vi "PicoLog_DATA.vi"(0 "noOfChannels":i16, 1 "handle":i16, 2 "sampleInterval_ms":dbl) -> (3 "handle":i16, 4 "P4":dbl[](graph), 5 "P5":dbl[](graph), 6 "Waveform Graph 3":dynamicdata(graph), 7 "P1":dbl[](graph), 8 "P2":dbl[](graph), 9 "P3":dbl[](graph))   [LabVIEW 2014]
uses:
  picohrdl.dll
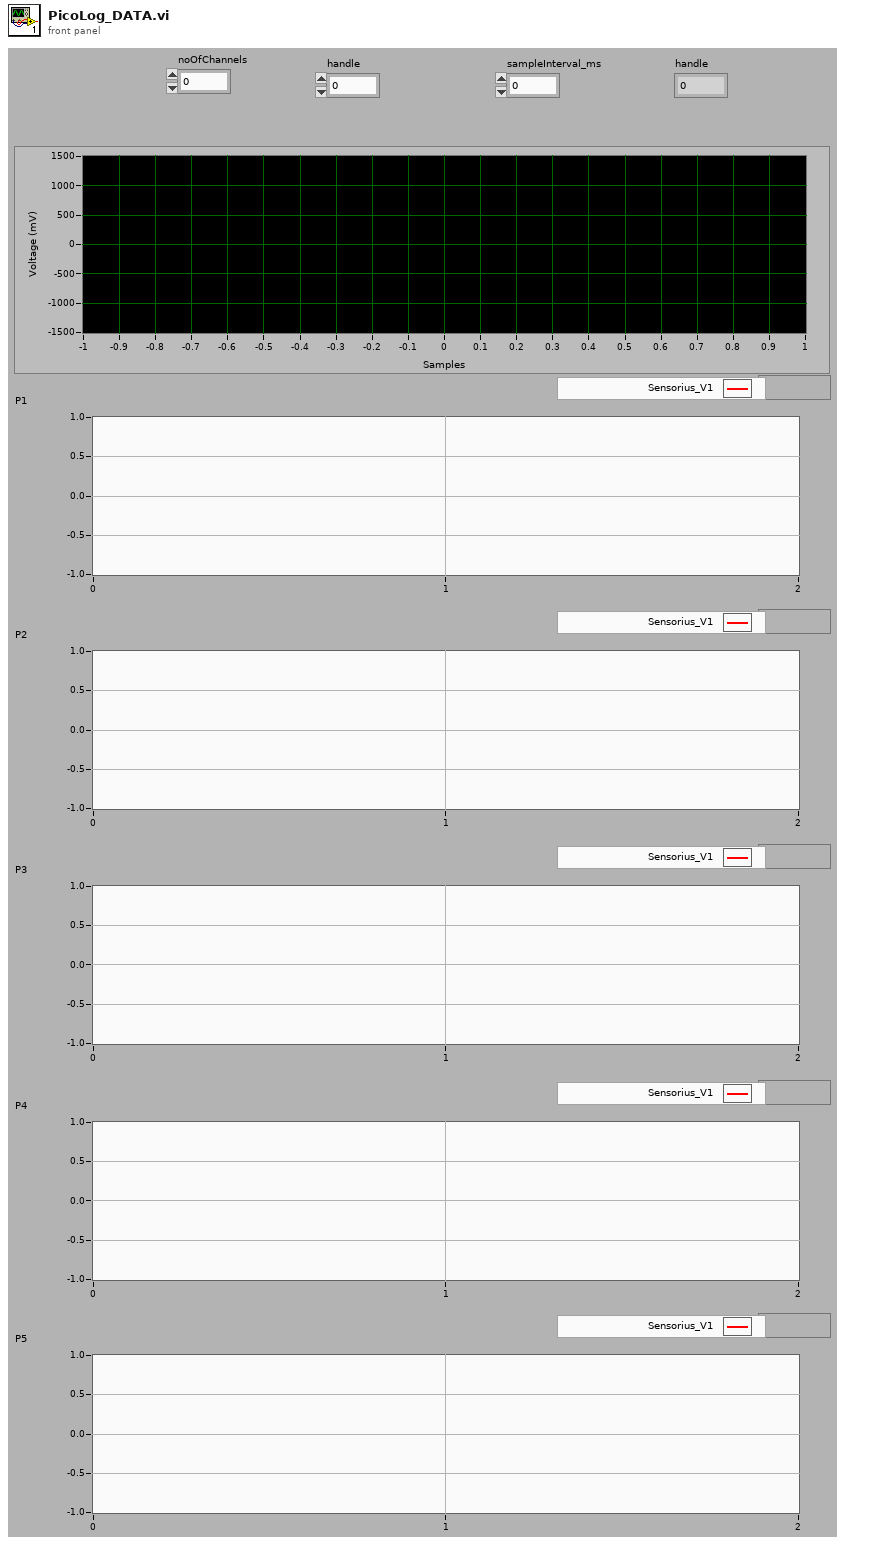
[diagram p1: front panel]
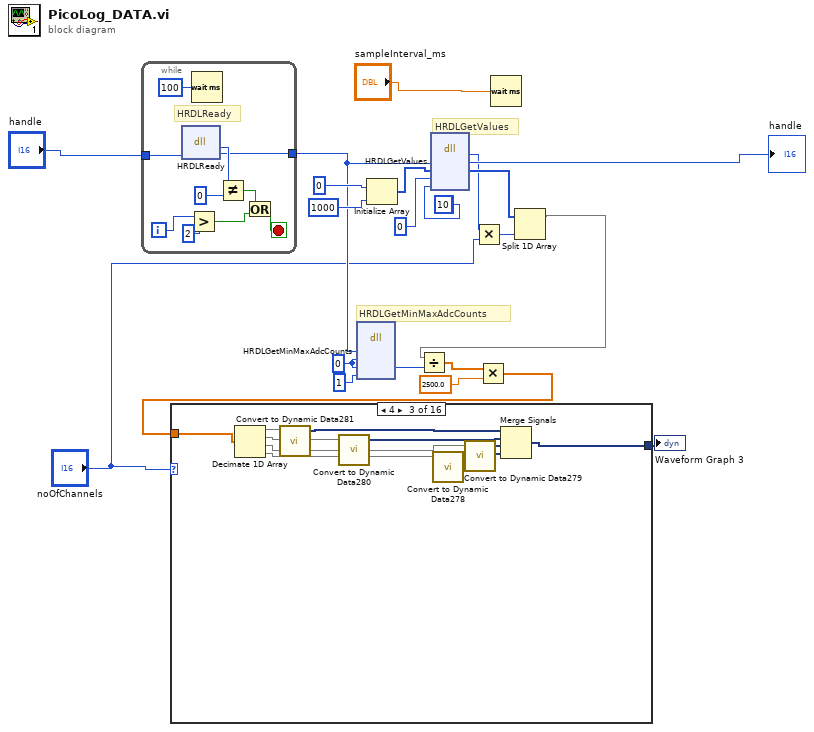
[diagram p0: block diagram]
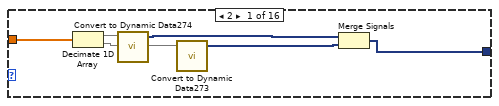
[diagram p2: hidden frame]
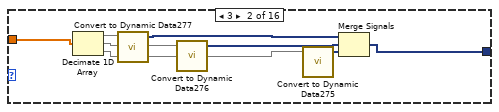
[diagram p3: hidden frame]
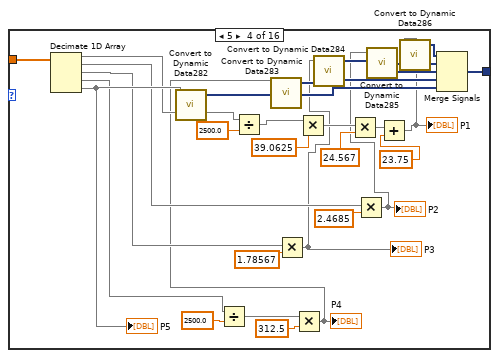
[diagram p4: hidden frame]
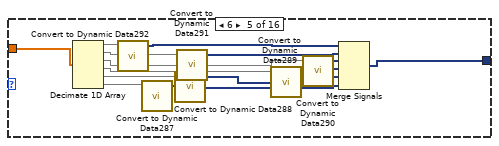
[diagram p5: hidden frame]
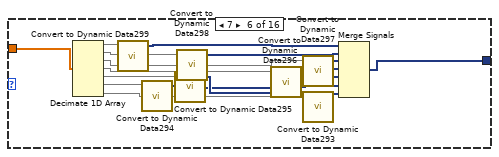
[diagram p6: hidden frame]
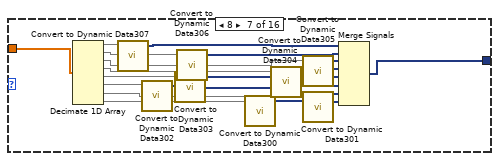
[diagram p7: hidden frame]
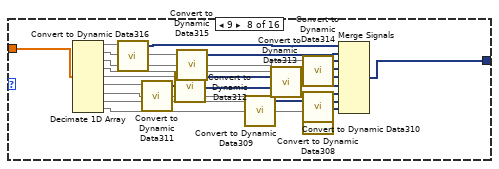
[diagram p8: hidden frame]
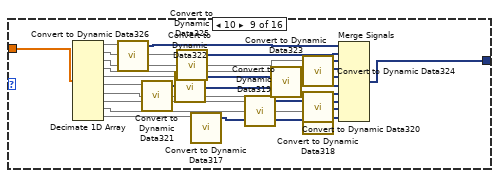
[diagram p9: hidden frame]
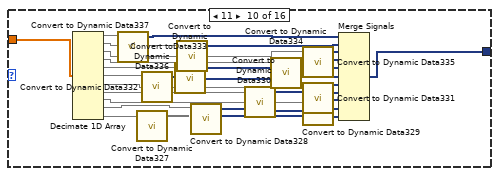
[diagram p10: hidden frame]
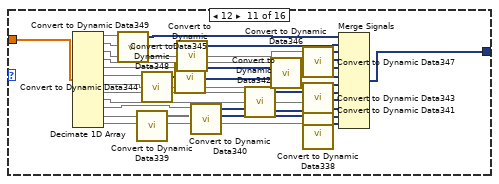
[diagram p11: hidden frame]
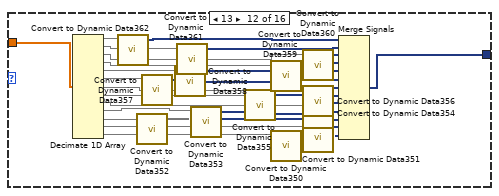
[diagram p12: hidden frame]
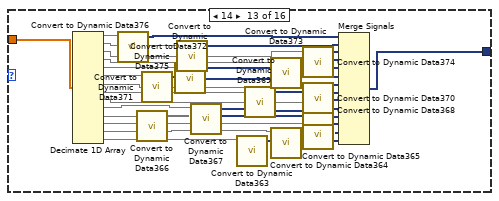
[diagram p13: hidden frame]
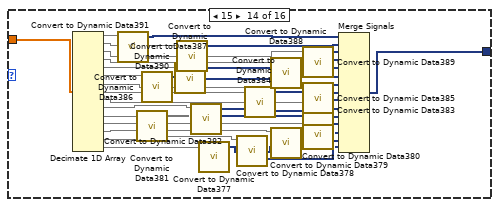
[diagram p14: hidden frame]
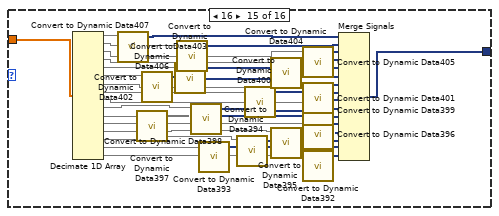
[diagram p15: hidden frame]
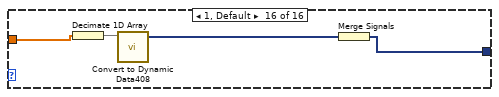
[diagram p16: hidden frame]
diagram:
  w14 = 0 ("maxAdc")
  (unwired) 10 ("noOfValues")
  # "HRDLGetMinMaxAdcCounts"
  # "HRDLGetValues"
  n1 = while {
    tunnel: "handle" -> [w29]
    tunnel: [w28] -> w6
    i -> [w26]
    stop <- w24 stop-if-true
    # "HRDLReady"
    n2 = dll-call lib="PicoHRDL.dll" fn="HRDLReady"("handle"=w29) -> ("ready"=w31:i16, "handle"=w28:i16)  [unwired: 3 in, 2 out]
    n3 = Greater?(x=w26, y=2) -> (0:w22:bool)
    n4 = Wait (ms)(milliseconds to wait=u32 100) -> ()  [unwired: 1 out]
    n5 = Not Equal?(x=w31, y=i16 0) -> (x != y?=w23:bool)
    n6 = Or(x=w23, y=w22) -> (x .or. y?=w24:bool)
  }
  n7 = dll-call lib="PicoHRDL.dll" fn="HRDLGetMinMaxAdcCounts"("handle"=w6, "minAdc"=w14, "maxAdc"=w14, "channel"=i16 1) -> ("maxAdc"=w9:i32)  [unwired: 7 in, 2 out]
  n8 = Initialize Array(0 ("element"), 1000 ("dimension size")) -> (w21:i32[])
  n9 = dll-call lib="PicoHRDL.dll" fn="HRDLGetValues"("handle"=w6, "values"=w21, "overflow"=i16 0, "noOfValues"=10) -> ("noValuesPerChan"=w10:i32, "handle"=→"handle":i16, "values"=w12:i32[])  [unwired: 5 in, 2 out]
  n10 = Multiply(x=w10, y="noOfChannels") -> (x*y=w11:i32)
  n11 = Wait (ms)(milliseconds to wait="sampleInterval_ms") -> ()  [unwired: 1 out]
  n12 = Split 1D Array(array=w12, index=w11) -> (first subarray=w4:i32[])  [unwired: 1 out]
  n13 = Divide(x=w4, y=w9) -> (x/y=w13:dbl[])
  n14 = Multiply(x=w13, y=2500.0) -> (x*y=w3:dbl[])
  n15 = case shown="4" "noOfChannels" {
    tunnel: [w33 w41 w51 w81 w93 w109 w127 w147 w169 w193 w219 w247 w277 w309 w343 w349] -> w5
    tunnel: w3 -> [w32 w40 w50 w80 w92 w108 w126 w146 w168 w192 w218 w246 w276 w308 w342 w348]
    frame 2 {
      n16 = Decimate 1D Array(w32) -> (w34:dbl[], w36:dbl[])
      n17 = call "Convert to Dynamic Data274"("Array"=w34) -> ("Dynamic Data Type"=w35:dynamicdata)  [unwired: 3 in]
      n18 = call "Convert to Dynamic Data273"("Array"=w36) -> ("Dynamic Data Type"=w37:dynamicdata)  [unwired: 3 in]
      n19 = Merge Signals(w35, w37) -> (w33:dynamicdata)
    }
    frame 3 {
      n20 = Decimate 1D Array(w40) -> (w42:dbl[], w44:dbl[], w38:dbl[])
      n21 = call "Convert to Dynamic Data277"("Array"=w42) -> ("Dynamic Data Type"=w43:dynamicdata)  [unwired: 3 in]
      n22 = call "Convert to Dynamic Data276"("Array"=w44) -> ("Dynamic Data Type"=w45:dynamicdata)  [unwired: 3 in]
      n23 = call "Convert to Dynamic Data275"("Array"=w38) -> ("Dynamic Data Type"=w39:dynamicdata)  [unwired: 3 in]
      n24 = Merge Signals(w43, w45, w39) -> (w41:dynamicdata)
    }
    frame 4 {
      n25 = Decimate 1D Array(w50) -> (w52:dbl[], w54:dbl[], w49:dbl[], w47:dbl[])
      n26 = call "Convert to Dynamic Data281"("Array"=w52) -> ("Dynamic Data Type"=w53:dynamicdata)  [unwired: 3 in]
      n27 = call "Convert to Dynamic Data280"("Array"=w54) -> ("Dynamic Data Type"=w55:dynamicdata)  [unwired: 3 in]
      n28 = call "Convert to Dynamic Data278"("Array"=w47) -> ("Dynamic Data Type"=w46:dynamicdata)  [unwired: 3 in]
      n29 = call "Convert to Dynamic Data279"("Array"=w49) -> ("Dynamic Data Type"=w48:dynamicdata)  [unwired: 3 in]
      n30 = Merge Signals(w53, w55, w48, w46) -> (w51:dynamicdata)
    }
    frame 5 {
      n31 = Decimate 1D Array(w80) -> (w75:dbl[], w62:dbl[], w60:dbl[], w72:dbl[], w76:dbl[])
      "P5" <- w76
      n32 = call "Convert to Dynamic Data282"("Array"=w76) -> ("Dynamic Data Type"=w77:dynamicdata)  [unwired: 3 in]
      n33 = Divide(x=w72, y=2500.0) -> (x/y=w73:dbl[])
      n34 = Divide(x=w75, y=2500.0) -> (x/y=w74:dbl[])
      n35 = Multiply(x=w60, y=1.78567) -> (x*y=w57:dbl[])
      "P3" <- w57
      n36 = Multiply(x=w73, y=312.5) -> (x*y=w56:dbl[])
      "P4" <- w56
      n37 = call "Convert to Dynamic Data283"("Array"=w56) -> ("Dynamic Data Type"=w78:dynamicdata)  [unwired: 3 in]
      n38 = Multiply(x=w74, y=39.0625) -> (x*y=w67:dbl[])
      n39 = call "Convert to Dynamic Data284"("Array"=w57) -> ("Dynamic Data Type"=w79:dynamicdata)  [unwired: 3 in]
      n40 = Multiply(x=w67, y=24.567) -> (x*y=w64:dbl[])
      n41 = Multiply(x=w62, y=2.4685) -> (x*y=w58:dbl[])
      "P2" <- w58
      n42 = call "Convert to Dynamic Data285"("Array"=w58) -> ("Dynamic Data Type"=w83:dynamicdata)  [unwired: 3 in]
      n43 = Add(x=w64, y=23.75) -> (x+y=w59:dbl[])
      "P1" <- w59
      n44 = call "Convert to Dynamic Data286"("Array"=w59) -> ("Dynamic Data Type"=w82:dynamicdata)  [unwired: 3 in]
      n45 = Merge Signals(w82, w83, w79, w78, w77) -> (w81:dynamicdata)
    }
    frame 6 {
      n46 = Decimate 1D Array(w92) -> (w94:dbl[], w96:dbl[], w91:dbl[], w89:dbl[], w87:dbl[], w85:dbl[])
      n47 = call "Convert to Dynamic Data292"("Array"=w94) -> ("Dynamic Data Type"=w95:dynamicdata)  [unwired: 3 in]
      n48 = call "Convert to Dynamic Data287"("Array"=w85) -> ("Dynamic Data Type"=w84:dynamicdata)  [unwired: 3 in]
      n49 = call "Convert to Dynamic Data288"("Array"=w87) -> ("Dynamic Data Type"=w86:dynamicdata)  [unwired: 3 in]
      n50 = call "Convert to Dynamic Data291"("Array"=w96) -> ("Dynamic Data Type"=w97:dynamicdata)  [unwired: 3 in]
      n51 = call "Convert to Dynamic Data289"("Array"=w89) -> ("Dynamic Data Type"=w88:dynamicdata)  [unwired: 3 in]
      n52 = call "Convert to Dynamic Data290"("Array"=w91) -> ("Dynamic Data Type"=w90:dynamicdata)  [unwired: 3 in]
      n53 = Merge Signals(w95, w97, w90, w88, w86, w84) -> (w93:dynamicdata)
    }
    frame 7 {
      n54 = Decimate 1D Array(w108) -> (w110:dbl[], w112:dbl[], w107:dbl[], w105:dbl[], w103:dbl[], w101:dbl[], w99:dbl[])
      n55 = call "Convert to Dynamic Data299"("Array"=w110) -> ("Dynamic Data Type"=w111:dynamicdata)  [unwired: 3 in]
      n56 = call "Convert to Dynamic Data294"("Array"=w101) -> ("Dynamic Data Type"=w100:dynamicdata)  [unwired: 3 in]
      n57 = call "Convert to Dynamic Data295"("Array"=w103) -> ("Dynamic Data Type"=w102:dynamicdata)  [unwired: 3 in]
      n58 = call "Convert to Dynamic Data298"("Array"=w112) -> ("Dynamic Data Type"=w113:dynamicdata)  [unwired: 3 in]
      n59 = call "Convert to Dynamic Data296"("Array"=w105) -> ("Dynamic Data Type"=w104:dynamicdata)  [unwired: 3 in]
      n60 = call "Convert to Dynamic Data297"("Array"=w107) -> ("Dynamic Data Type"=w106:dynamicdata)  [unwired: 3 in]
      n61 = call "Convert to Dynamic Data293"("Array"=w99) -> ("Dynamic Data Type"=w98:dynamicdata)  [unwired: 3 in]
      n62 = Merge Signals(w111, w113, w106, w104, w102, w100, w98) -> (w109:dynamicdata)
    }
    frame 8 {
      n63 = Decimate 1D Array(w126) -> (w128:dbl[], w130:dbl[], w125:dbl[], w123:dbl[], w121:dbl[], w119:dbl[], w117:dbl[], w115:dbl[])
      n64 = call "Convert to Dynamic Data307"("Array"=w128) -> ("Dynamic Data Type"=w129:dynamicdata)  [unwired: 3 in]
      n65 = call "Convert to Dynamic Data302"("Array"=w119) -> ("Dynamic Data Type"=w118:dynamicdata)  [unwired: 3 in]
      n66 = call "Convert to Dynamic Data303"("Array"=w121) -> ("Dynamic Data Type"=w120:dynamicdata)  [unwired: 3 in]
      n67 = call "Convert to Dynamic Data306"("Array"=w130) -> ("Dynamic Data Type"=w131:dynamicdata)  [unwired: 3 in]
      n68 = call "Convert to Dynamic Data300"("Array"=w115) -> ("Dynamic Data Type"=w114:dynamicdata)  [unwired: 3 in]
      n69 = call "Convert to Dynamic Data304"("Array"=w123) -> ("Dynamic Data Type"=w122:dynamicdata)  [unwired: 3 in]
      n70 = call "Convert to Dynamic Data305"("Array"=w125) -> ("Dynamic Data Type"=w124:dynamicdata)  [unwired: 3 in]
      n71 = call "Convert to Dynamic Data301"("Array"=w117) -> ("Dynamic Data Type"=w116:dynamicdata)  [unwired: 3 in]
      n72 = Merge Signals(w129, w131, w124, w122, w120, w118, w116, w114) -> (w127:dynamicdata)
    }
    frame 9 {
      n73 = Decimate 1D Array(w146) -> (w148:dbl[], w150:dbl[], w145:dbl[], w143:dbl[], w141:dbl[], w139:dbl[], w137:dbl[], w135:dbl[], w133:dbl[])
      n74 = call "Convert to Dynamic Data316"("Array"=w148) -> ("Dynamic Data Type"=w149:dynamicdata)  [unwired: 3 in]
      n75 = call "Convert to Dynamic Data311"("Array"=w139) -> ("Dynamic Data Type"=w138:dynamicdata)  [unwired: 3 in]
      n76 = call "Convert to Dynamic Data312"("Array"=w141) -> ("Dynamic Data Type"=w140:dynamicdata)  [unwired: 3 in]
      n77 = call "Convert to Dynamic Data315"("Array"=w150) -> ("Dynamic Data Type"=w151:dynamicdata)  [unwired: 3 in]
      n78 = call "Convert to Dynamic Data309"("Array"=w135) -> ("Dynamic Data Type"=w134:dynamicdata)  [unwired: 3 in]
      n79 = call "Convert to Dynamic Data313"("Array"=w143) -> ("Dynamic Data Type"=w142:dynamicdata)  [unwired: 3 in]
      n80 = call "Convert to Dynamic Data314"("Array"=w145) -> ("Dynamic Data Type"=w144:dynamicdata)  [unwired: 3 in]
      n81 = call "Convert to Dynamic Data310"("Array"=w137) -> ("Dynamic Data Type"=w136:dynamicdata)  [unwired: 3 in]
      n82 = call "Convert to Dynamic Data308"("Array"=w133) -> ("Dynamic Data Type"=w132:dynamicdata)  [unwired: 3 in]
      n83 = Merge Signals(w149, w151, w144, w142, w140, w138, w136, w134, w132) -> (w147:dynamicdata)
    }
    frame 10 {
      n84 = Decimate 1D Array(w168) -> (w170:dbl[], w172:dbl[], w167:dbl[], w165:dbl[], w163:dbl[], w161:dbl[], w159:dbl[], w157:dbl[], w155:dbl[], w153:dbl[])
      n85 = call "Convert to Dynamic Data326"("Array"=w170) -> ("Dynamic Data Type"=w171:dynamicdata)  [unwired: 3 in]
      n86 = call "Convert to Dynamic Data321"("Array"=w161) -> ("Dynamic Data Type"=w160:dynamicdata)  [unwired: 3 in]
      n87 = call "Convert to Dynamic Data322"("Array"=w163) -> ("Dynamic Data Type"=w162:dynamicdata)  [unwired: 3 in]
      n88 = call "Convert to Dynamic Data325"("Array"=w172) -> ("Dynamic Data Type"=w173:dynamicdata)  [unwired: 3 in]
      n89 = call "Convert to Dynamic Data317"("Array"=w153) -> ("Dynamic Data Type"=w152:dynamicdata)  [unwired: 3 in]
      n90 = call "Convert to Dynamic Data319"("Array"=w157) -> ("Dynamic Data Type"=w156:dynamicdata)  [unwired: 3 in]
      n91 = call "Convert to Dynamic Data323"("Array"=w165) -> ("Dynamic Data Type"=w164:dynamicdata)  [unwired: 3 in]
      n92 = call "Convert to Dynamic Data324"("Array"=w167) -> ("Dynamic Data Type"=w166:dynamicdata)  [unwired: 3 in]
      n93 = call "Convert to Dynamic Data320"("Array"=w159) -> ("Dynamic Data Type"=w158:dynamicdata)  [unwired: 3 in]
      n94 = call "Convert to Dynamic Data318"("Array"=w155) -> ("Dynamic Data Type"=w154:dynamicdata)  [unwired: 3 in]
      n95 = Merge Signals(w171, w173, w166, w164, w162, w160, w158, w156, w154, w152) -> (w169:dynamicdata)
    }
    frame 11 {
      n96 = Decimate 1D Array(w192) -> (w194:dbl[], w196:dbl[], w191:dbl[], w189:dbl[], w187:dbl[], w185:dbl[], w183:dbl[], w181:dbl[], w179:dbl[], w177:dbl[], w175:dbl[])
      n97 = call "Convert to Dynamic Data337"("Array"=w194) -> ("Dynamic Data Type"=w195:dynamicdata)  [unwired: 3 in]
      n98 = call "Convert to Dynamic Data327"("Array"=w175) -> ("Dynamic Data Type"=w174:dynamicdata)  [unwired: 3 in]
      n99 = call "Convert to Dynamic Data332"("Array"=w185) -> ("Dynamic Data Type"=w184:dynamicdata)  [unwired: 3 in]
      n100 = call "Convert to Dynamic Data333"("Array"=w187) -> ("Dynamic Data Type"=w186:dynamicdata)  [unwired: 3 in]
      n101 = call "Convert to Dynamic Data336"("Array"=w196) -> ("Dynamic Data Type"=w197:dynamicdata)  [unwired: 3 in]
      n102 = call "Convert to Dynamic Data328"("Array"=w177) -> ("Dynamic Data Type"=w176:dynamicdata)  [unwired: 3 in]
      n103 = call "Convert to Dynamic Data330"("Array"=w181) -> ("Dynamic Data Type"=w180:dynamicdata)  [unwired: 3 in]
      n104 = call "Convert to Dynamic Data334"("Array"=w189) -> ("Dynamic Data Type"=w188:dynamicdata)  [unwired: 3 in]
      n105 = call "Convert to Dynamic Data335"("Array"=w191) -> ("Dynamic Data Type"=w190:dynamicdata)  [unwired: 3 in]
      n106 = call "Convert to Dynamic Data331"("Array"=w183) -> ("Dynamic Data Type"=w182:dynamicdata)  [unwired: 3 in]
      n107 = call "Convert to Dynamic Data329"("Array"=w179) -> ("Dynamic Data Type"=w178:dynamicdata)  [unwired: 3 in]
      n108 = Merge Signals(w195, w197, w190, w188, w186, w184, w182, w180, w178, w176, w174) -> (w193:dynamicdata)
    }
    frame 12 {
      n109 = Decimate 1D Array(w218) -> (w220:dbl[], w222:dbl[], w217:dbl[], w215:dbl[], w213:dbl[], w211:dbl[], w209:dbl[], w207:dbl[], w205:dbl[], w203:dbl[], w201:dbl[], w199:dbl[])
      n110 = call "Convert to Dynamic Data349"("Array"=w220) -> ("Dynamic Data Type"=w221:dynamicdata)  [unwired: 3 in]
      n111 = call "Convert to Dynamic Data339"("Array"=w201) -> ("Dynamic Data Type"=w200:dynamicdata)  [unwired: 3 in]
      n112 = call "Convert to Dynamic Data344"("Array"=w211) -> ("Dynamic Data Type"=w210:dynamicdata)  [unwired: 3 in]
      n113 = call "Convert to Dynamic Data345"("Array"=w213) -> ("Dynamic Data Type"=w212:dynamicdata)  [unwired: 3 in]
      n114 = call "Convert to Dynamic Data348"("Array"=w222) -> ("Dynamic Data Type"=w223:dynamicdata)  [unwired: 3 in]
      n115 = call "Convert to Dynamic Data340"("Array"=w203) -> ("Dynamic Data Type"=w202:dynamicdata)  [unwired: 3 in]
      n116 = call "Convert to Dynamic Data342"("Array"=w207) -> ("Dynamic Data Type"=w206:dynamicdata)  [unwired: 3 in]
      n117 = call "Convert to Dynamic Data346"("Array"=w215) -> ("Dynamic Data Type"=w214:dynamicdata)  [unwired: 3 in]
      n118 = call "Convert to Dynamic Data347"("Array"=w217) -> ("Dynamic Data Type"=w216:dynamicdata)  [unwired: 3 in]
      n119 = call "Convert to Dynamic Data343"("Array"=w209) -> ("Dynamic Data Type"=w208:dynamicdata)  [unwired: 3 in]
      n120 = call "Convert to Dynamic Data341"("Array"=w205) -> ("Dynamic Data Type"=w204:dynamicdata)  [unwired: 3 in]
      n121 = call "Convert to Dynamic Data338"("Array"=w199) -> ("Dynamic Data Type"=w198:dynamicdata)  [unwired: 3 in]
      n122 = Merge Signals(w221, w223, w216, w214, w212, w210, w208, w206, w204, w202, w200, w198) -> (w219:dynamicdata)
    }
    frame 13 {
      n123 = Decimate 1D Array(w246) -> (w248:dbl[], w250:dbl[], w245:dbl[], w243:dbl[], w241:dbl[], w239:dbl[], w237:dbl[], w235:dbl[], w233:dbl[], w231:dbl[], w229:dbl[], w227:dbl[], w225:dbl[])
      n124 = call "Convert to Dynamic Data362"("Array"=w248) -> ("Dynamic Data Type"=w249:dynamicdata)  [unwired: 3 in]
      n125 = call "Convert to Dynamic Data352"("Array"=w229) -> ("Dynamic Data Type"=w228:dynamicdata)  [unwired: 3 in]
      n126 = call "Convert to Dynamic Data357"("Array"=w239) -> ("Dynamic Data Type"=w238:dynamicdata)  [unwired: 3 in]
      n127 = call "Convert to Dynamic Data358"("Array"=w241) -> ("Dynamic Data Type"=w240:dynamicdata)  [unwired: 3 in]
      n128 = call "Convert to Dynamic Data361"("Array"=w250) -> ("Dynamic Data Type"=w251:dynamicdata)  [unwired: 3 in]
      n129 = call "Convert to Dynamic Data353"("Array"=w231) -> ("Dynamic Data Type"=w230:dynamicdata)  [unwired: 3 in]
      n130 = call "Convert to Dynamic Data355"("Array"=w235) -> ("Dynamic Data Type"=w234:dynamicdata)  [unwired: 3 in]
      n131 = call "Convert to Dynamic Data359"("Array"=w243) -> ("Dynamic Data Type"=w242:dynamicdata)  [unwired: 3 in]
      n132 = call "Convert to Dynamic Data350"("Array"=w225) -> ("Dynamic Data Type"=w224:dynamicdata)  [unwired: 3 in]
      n133 = call "Convert to Dynamic Data360"("Array"=w245) -> ("Dynamic Data Type"=w244:dynamicdata)  [unwired: 3 in]
      n134 = call "Convert to Dynamic Data356"("Array"=w237) -> ("Dynamic Data Type"=w236:dynamicdata)  [unwired: 3 in]
      n135 = call "Convert to Dynamic Data354"("Array"=w233) -> ("Dynamic Data Type"=w232:dynamicdata)  [unwired: 3 in]
      n136 = call "Convert to Dynamic Data351"("Array"=w227) -> ("Dynamic Data Type"=w226:dynamicdata)  [unwired: 3 in]
      n137 = Merge Signals(w249, w251, w244, w242, w240, w238, w236, w234, w232, w230, w228, w226, w224) -> (w247:dynamicdata)
    }
    frame 14 {
      n138 = Decimate 1D Array(w276) -> (w278:dbl[], w280:dbl[], w275:dbl[], w273:dbl[], w271:dbl[], w269:dbl[], w267:dbl[], w265:dbl[], w263:dbl[], w261:dbl[], w259:dbl[], w257:dbl[], w255:dbl[], w253:dbl[])
      n139 = call "Convert to Dynamic Data376"("Array"=w278) -> ("Dynamic Data Type"=w279:dynamicdata)  [unwired: 3 in]
      n140 = call "Convert to Dynamic Data366"("Array"=w259) -> ("Dynamic Data Type"=w258:dynamicdata)  [unwired: 3 in]
      n141 = call "Convert to Dynamic Data371"("Array"=w269) -> ("Dynamic Data Type"=w268:dynamicdata)  [unwired: 3 in]
      n142 = call "Convert to Dynamic Data372"("Array"=w271) -> ("Dynamic Data Type"=w270:dynamicdata)  [unwired: 3 in]
      n143 = call "Convert to Dynamic Data375"("Array"=w280) -> ("Dynamic Data Type"=w281:dynamicdata)  [unwired: 3 in]
      n144 = call "Convert to Dynamic Data367"("Array"=w261) -> ("Dynamic Data Type"=w260:dynamicdata)  [unwired: 3 in]
      n145 = call "Convert to Dynamic Data363"("Array"=w253) -> ("Dynamic Data Type"=w252:dynamicdata)  [unwired: 3 in]
      n146 = call "Convert to Dynamic Data369"("Array"=w265) -> ("Dynamic Data Type"=w264:dynamicdata)  [unwired: 3 in]
      n147 = call "Convert to Dynamic Data373"("Array"=w273) -> ("Dynamic Data Type"=w272:dynamicdata)  [unwired: 3 in]
      n148 = call "Convert to Dynamic Data364"("Array"=w255) -> ("Dynamic Data Type"=w254:dynamicdata)  [unwired: 3 in]
      n149 = call "Convert to Dynamic Data374"("Array"=w275) -> ("Dynamic Data Type"=w274:dynamicdata)  [unwired: 3 in]
      n150 = call "Convert to Dynamic Data370"("Array"=w267) -> ("Dynamic Data Type"=w266:dynamicdata)  [unwired: 3 in]
      n151 = call "Convert to Dynamic Data368"("Array"=w263) -> ("Dynamic Data Type"=w262:dynamicdata)  [unwired: 3 in]
      n152 = call "Convert to Dynamic Data365"("Array"=w257) -> ("Dynamic Data Type"=w256:dynamicdata)  [unwired: 3 in]
      n153 = Merge Signals(w279, w281, w274, w272, w270, w268, w266, w264, w262, w260, w258, w256, w254, w252) -> (w277:dynamicdata)
    }
    frame 15 {
      n154 = Decimate 1D Array(w308) -> (w310:dbl[], w312:dbl[], w307:dbl[], w305:dbl[], w303:dbl[], w301:dbl[], w299:dbl[], w297:dbl[], w295:dbl[], w293:dbl[], w291:dbl[], w289:dbl[], w287:dbl[], w285:dbl[], w283:dbl[])
      n155 = call "Convert to Dynamic Data391"("Array"=w310) -> ("Dynamic Data Type"=w311:dynamicdata)  [unwired: 3 in]
      n156 = call "Convert to Dynamic Data381"("Array"=w291) -> ("Dynamic Data Type"=w290:dynamicdata)  [unwired: 3 in]
      n157 = call "Convert to Dynamic Data386"("Array"=w301) -> ("Dynamic Data Type"=w300:dynamicdata)  [unwired: 3 in]
      n158 = call "Convert to Dynamic Data387"("Array"=w303) -> ("Dynamic Data Type"=w302:dynamicdata)  [unwired: 3 in]
      n159 = call "Convert to Dynamic Data390"("Array"=w312) -> ("Dynamic Data Type"=w313:dynamicdata)  [unwired: 3 in]
      n160 = call "Convert to Dynamic Data382"("Array"=w293) -> ("Dynamic Data Type"=w292:dynamicdata)  [unwired: 3 in]
      n161 = call "Convert to Dynamic Data377"("Array"=w283) -> ("Dynamic Data Type"=w282:dynamicdata)  [unwired: 3 in]
      n162 = call "Convert to Dynamic Data378"("Array"=w285) -> ("Dynamic Data Type"=w284:dynamicdata)  [unwired: 3 in]
      n163 = call "Convert to Dynamic Data384"("Array"=w297) -> ("Dynamic Data Type"=w296:dynamicdata)  [unwired: 3 in]
      n164 = call "Convert to Dynamic Data388"("Array"=w305) -> ("Dynamic Data Type"=w304:dynamicdata)  [unwired: 3 in]
      n165 = call "Convert to Dynamic Data379"("Array"=w287) -> ("Dynamic Data Type"=w286:dynamicdata)  [unwired: 3 in]
      n166 = call "Convert to Dynamic Data389"("Array"=w307) -> ("Dynamic Data Type"=w306:dynamicdata)  [unwired: 3 in]
      n167 = call "Convert to Dynamic Data385"("Array"=w299) -> ("Dynamic Data Type"=w298:dynamicdata)  [unwired: 3 in]
      n168 = call "Convert to Dynamic Data383"("Array"=w295) -> ("Dynamic Data Type"=w294:dynamicdata)  [unwired: 3 in]
      n169 = call "Convert to Dynamic Data380"("Array"=w289) -> ("Dynamic Data Type"=w288:dynamicdata)  [unwired: 3 in]
      n170 = Merge Signals(w311, w313, w306, w304, w302, w300, w298, w296, w294, w292, w290, w288, w286, w284, w282) -> (w309:dynamicdata)
    }
    frame 16 {
      n171 = Decimate 1D Array(w342) -> (w344:dbl[], w346:dbl[], w341:dbl[], w339:dbl[], w337:dbl[], w335:dbl[], w333:dbl[], w331:dbl[], w329:dbl[], w327:dbl[], w325:dbl[], w323:dbl[], w321:dbl[], w319:dbl[], w317:dbl[], w315:dbl[])
      n172 = call "Convert to Dynamic Data407"("Array"=w344) -> ("Dynamic Data Type"=w345:dynamicdata)  [unwired: 3 in]
      n173 = call "Convert to Dynamic Data397"("Array"=w325) -> ("Dynamic Data Type"=w324:dynamicdata)  [unwired: 3 in]
      n174 = call "Convert to Dynamic Data402"("Array"=w335) -> ("Dynamic Data Type"=w334:dynamicdata)  [unwired: 3 in]
      n175 = call "Convert to Dynamic Data403"("Array"=w337) -> ("Dynamic Data Type"=w336:dynamicdata)  [unwired: 3 in]
      n176 = call "Convert to Dynamic Data406"("Array"=w346) -> ("Dynamic Data Type"=w347:dynamicdata)  [unwired: 3 in]
      n177 = call "Convert to Dynamic Data398"("Array"=w327) -> ("Dynamic Data Type"=w326:dynamicdata)  [unwired: 3 in]
      n178 = call "Convert to Dynamic Data393"("Array"=w317) -> ("Dynamic Data Type"=w316:dynamicdata)  [unwired: 3 in]
      n179 = call "Convert to Dynamic Data394"("Array"=w319) -> ("Dynamic Data Type"=w318:dynamicdata)  [unwired: 3 in]
      n180 = call "Convert to Dynamic Data400"("Array"=w331) -> ("Dynamic Data Type"=w330:dynamicdata)  [unwired: 3 in]
      n181 = call "Convert to Dynamic Data404"("Array"=w339) -> ("Dynamic Data Type"=w338:dynamicdata)  [unwired: 3 in]
      n182 = call "Convert to Dynamic Data395"("Array"=w321) -> ("Dynamic Data Type"=w320:dynamicdata)  [unwired: 3 in]
      n183 = call "Convert to Dynamic Data405"("Array"=w341) -> ("Dynamic Data Type"=w340:dynamicdata)  [unwired: 3 in]
      n184 = call "Convert to Dynamic Data401"("Array"=w333) -> ("Dynamic Data Type"=w332:dynamicdata)  [unwired: 3 in]
      n185 = call "Convert to Dynamic Data399"("Array"=w329) -> ("Dynamic Data Type"=w328:dynamicdata)  [unwired: 3 in]
      n186 = call "Convert to Dynamic Data396"("Array"=w323) -> ("Dynamic Data Type"=w322:dynamicdata)  [unwired: 3 in]
      n187 = call "Convert to Dynamic Data392"("Array"=w315) -> ("Dynamic Data Type"=w314:dynamicdata)  [unwired: 3 in]
      n188 = Merge Signals(w345, w347, w340, w338, w336, w334, w332, w330, w328, w326, w324, w322, w320, w318, w316, w314) -> (w343:dynamicdata)
    }
    frame 1, Default {
      n189 = Decimate 1D Array(w348) -> (w350:dbl[])
      n190 = call "Convert to Dynamic Data408"("Array"=w350) -> ("Dynamic Data Type"=w351:dynamicdata)  [unwired: 3 in]
      n191 = Merge Signals(w351) -> (w349:dynamicdata)
    }
  }
  "Waveform Graph 3" <- w5
